vi "SnakeNextPosIndex.vi"(8 "Array 4":u16[][](array[numeric]), 9 "Snake Positions":cluster{"R":i32, "C":i32}[](array[cluster]), 10 "c":i32, 11 "r":i32) -> (0 "Array 5":u16[][](array[numeric]), 1 "Array 2":cluster{"R":i32, "C":i32}[](array[cluster]))   [LabVIEW 2014]
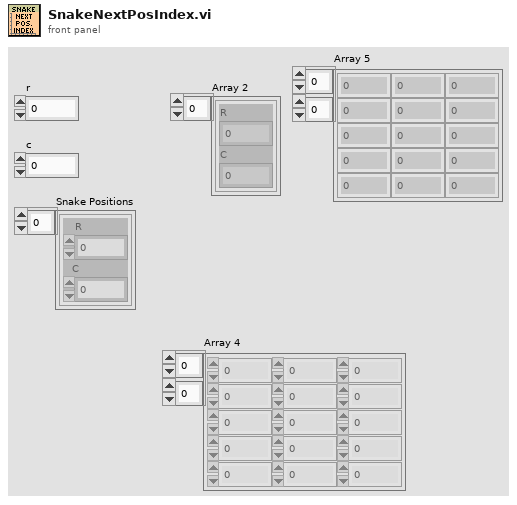
[diagram p1: front panel]
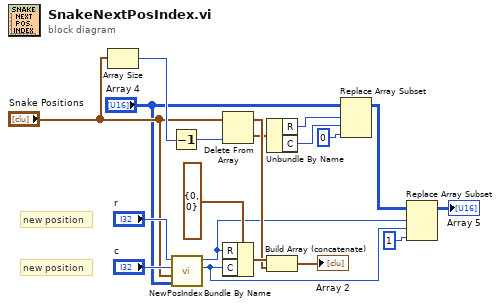
[diagram p0: block diagram]
diagram:
  # "new position"
  # "new position"
  n1 = Array Size(array="Snake Positions") -> (size(s)=w8:i32)
  n2 = Decrement(x=w8) -> (x-1=w9:i32)
  n3 = call "NewPosIndex.vi"("Array 4"="Array 4", "Snake Positions"="Snake Positions", "c"="c", "r"="r") -> ("newc"=w2:i32, "newr"=w3:i32)  [unwired: 6 in]
  n4 = Delete From Array(array="Snake Positions", index=w9) -> (deleted portion=w10:cluster{"R":i32, "C":i32}, array with subset deleted=w11:cluster{"R":i32, "C":i32}[])  [unwired: 1 in]
  n5 = Bundle By Name(cluster=cluster{"R":i32, "C":i32} {"R"=0, "C"=0}, "R"=w3, "C"=w2) -> (w13:cluster{"R":i32, "C":i32})
  n6 = Unbundle By Name(w10) -> ("R"=w14:i32, "C"=w15:i32)
  n7 = Build Array (concatenate)(w13, w11) -> (→"Array 2":cluster{"R":i32, "C":i32}[])
  n8 = Replace Array Subset(array="Array 4", new element=u16 0 ("new element/subarray"), index (row)=w14, index (col)=w15) -> (w19:u16[][])
  n9 = Replace Array Subset(array=w19, new element=u16 1 ("new element/subarray"), index (row)=w3, index (col)=w2) -> (→"Array 5":u16[][])
